vi "SineWave_testMyrioCounter.vi"() -> ()   [LabVIEW 2015]
uses:
  <vilib>/userdefined/High Color/nirio_resource_hc.ctl
  <vilib>/FPGAPlugInAG/myRIO-1900/niLvFpga_Open_myRIO-1900.vi
  <vilib>/FPGAPlugInAG/myRIO-1900/niLvFpga_Reset_myRIO-1900.vi
  <vilib>/rvi/interface/common/niFpgaWaitOnOcc.vi
  <vilib>/Utility/error.llb/Error Cluster From Error Code.vi
  <vilib>/rvi/errors/niLvFpgaAdjustHostInterfaceError.vi
  <vilib>/FPGAPlugInAG/myRIO-1900/niLvFpga_Run_myRIO-1900.vi
  <vilib>/FPGAPlugInAG/myRIO-1900/niLvFpga_Close_myRIO-1900.vi
  <vilib>/rvi/interface/nirviOpenFPGA/nirviOpenFPGA.xnode
  FPGA Bitfiles/MEMSPAMMyRIO_FPGATarget_testMyrioCounter_ZhKD5kzzM-g.lvbitx
  testMyrioCounter.vi
  <vilib>/rvi/interface/nirviMethod/nirviMethod.xnode
  <vilib>/rvi/interface/nirviReadWriteControl/nirviReadWriteControl.xnode
  <vilib>/rvi/interface/nirviCloseFPGA/nirviCloseFPGA.xnode
  <vilib>/Analysis/NI_AALPro.lvlib
  <vilib>/rvi/errors/niLvFpgaMergeErrorWithErrorCode.vi
  <vilib>/FPGAPlugInAG/myRIO-1900/niLvFpga_ConfigureFifo_myRIO-1900.vi
  <vilib>/FPGAPlugInAG/myRIO-1900/niLvFpga_WriteFifo_myRIO-1900.vi
  NiFpgaLv.dll
panel:
  out "Timed Out?":bool
  in  "stop":bool
  out "DA points":i32=440
  out "Bscan_Steps":u32[](graph)
  in  "Sample Num":u32=160
  in  "Range (V)":dbl=2.0 format="%0.2f"
  in  "Offset (V)":dbl format="%0.4f"
  in  "Phase0(deg)":dbl format="%0.2f"
  out "Vocie-coil Traj":i16[](graph)=[0, 16, 32, 48, 64, 80, 96, 111, 127, 142, 157, 171, 186, 200, 214, 228, 241, 254, 266, 278, 290, 301, 311, 322, 331, 341, 349, 357, 365, 372, 378, 384, 390, 394, 398, 402, 405, 407, 408, 409, 410, 409, 408, 407, 405, 402, 398, 394, 390, 384, 378, 372, 365, 357, 349, 341, 331, 322, 311, 301, 290, 278, 266, 254, 241, 228, 214, 200, 186, 171, 157, 142, 127, 111, 96, 80, 64, 48, 32, 16, 0, -16, -32, -48, -64, -80, -96, -111, -127, -142, -157, -171, -186, -200, -214, -228, -241, -254, -266, -278, -290, -301, -311, -322, -331, -341, -349, -357, -365, -372, -378, -384, -390, -394, -398, -402, -405, -407, -408, -409, -410, -409, -408, -407, -405, -402, -398, -394, -390, -384, -378, -372, -365, -357, -349, -341, -331, -322, -311, -301, -290, -278, -266, -254, -241, -228, -214, -200, -186, -171, -157, -142, -127, -111, -96, -80, -64, -48, -32, -16]
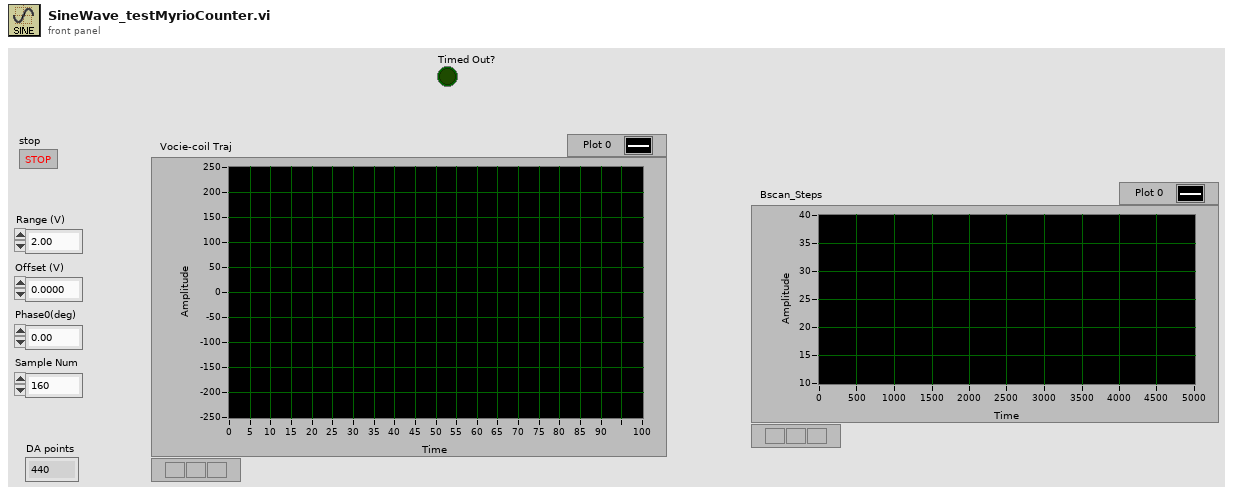
[diagram p1: front panel]
types:
  T1 = enum16{"sine", "cosine", "triangle", "square", "sawtooth", "increasing ramp", "decreasing ramp"}
  T2 = typedef "nirio_resource_hc.ctl" = tag
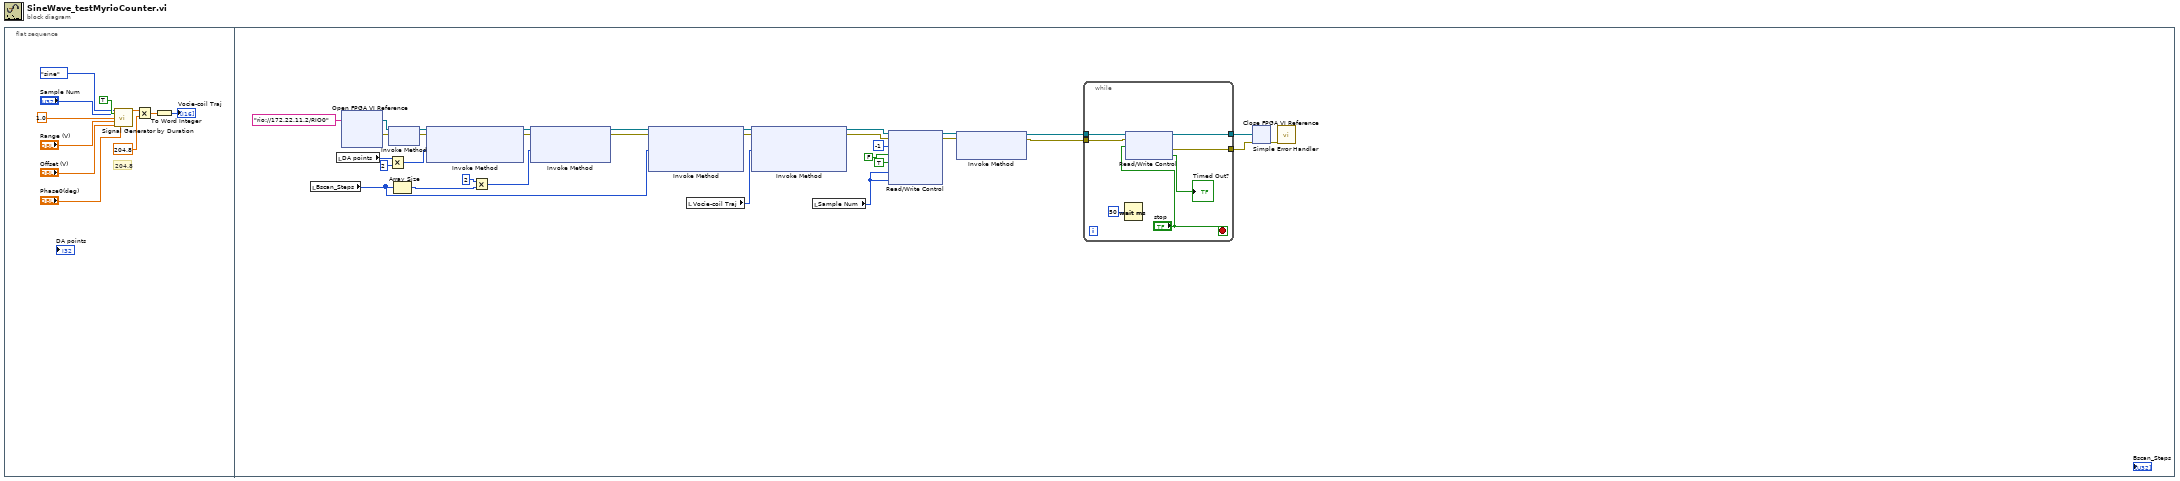
[diagram p0: block diagram]
diagram:
  n1 = flat-sequence {
    frame #0 {
      # "204.8"
      n2 = call <vilib>:"Signal Generator by Duration.vi"("signal type"=T1."sine", "reset phase"=TRUE, "# of samples"="Sample Num", "frequency"=1.0, "amplitude"="Range (V)", "dc offset"="Offset (V)", "phase in"="Phase0(deg)") -> ("signal"=w11:dbl[])  [unwired: 5 in, 3 out]
      n3 = Multiply(x=w11, y=204.8 ("frequency")) -> (x*y=w3:dbl[])
      n4 = To Word Integer(number=w3) -> (16bit integer=→"Vocie-coil Traj":i16[])
    }
    frame #1 {
      n5 = local read "Bscan_Steps"() -> (w40:u32[])
      n6 = local read "DA points"() -> (w15:i32)
      n7 = xnode "Open FPGA VI Reference"("resource name"=T2 "rio://172.22.11.2/RIO0") -> ("FPGA VI Reference Out"=w31:refnum<k20>, "error out"=w30:errorcluster)  [unwired: 1 in]
      n8 = xnode "Invoke Method"("FPGA VI Reference In"=w31, "error in"=w30) -> ("FPGA VI Reference Out"=w29:refnum<k20>, "error out"=w28:errorcluster)
      n9 = Multiply(x=w15, y=2) -> (x*y=w14:i32)
      n10 = Array Size(array=w40) -> (size(s)=w41:i32)
      n11 = xnode "Invoke Method"("FPGA VI Reference In"=w29, "error in"=w28, "Requested Depth"=w14) -> ("FPGA VI Reference Out"=w43:refnum<k20>, "error out"=w42:errorcluster)  [unwired: 1 out]
      n12 = Multiply(x=2, y=w41) -> (x*y=w37:i32)
      n13 = xnode "Invoke Method"("FPGA VI Reference In"=w43, "error in"=w42, "Requested Depth"=w37) -> ("FPGA VI Reference Out"=w34:refnum<k20>, "error out"=w33:errorcluster)  [unwired: 1 out]
      n14 = xnode "Invoke Method"("FPGA VI Reference In"=w34, "error in"=w33, "Data"=w40) -> ("FPGA VI Reference Out"=w35:refnum<k20>, "error out"=w36:errorcluster)  [unwired: 1 in, 1 out]
      n15 = local read "Vocie-coil Traj"() -> (w39:i16[])
      n16 = xnode "Invoke Method"("FPGA VI Reference In"=w35, "error in"=w36, "Data"=w39) -> ("FPGA VI Reference Out"=w27:refnum<k20>, "error out"=w24:errorcluster)  [unwired: 1 in, 1 out]
      n17 = local read "Sample Num"() -> (w12:u32)
      n18 = xnode "Read/Write Control"("FPGA VI Reference In"=w27, "error in"=w24, "FIFO_Timeout"=-1, "stop"=FALSE, "Sine"=TRUE, "VC_pt_in_fifo"=w12, "Trigperscan"=w12) -> ("FPGA VI Reference Out"=w25:refnum<k20>, "error out"=w23:errorcluster)
      n19 = xnode "Invoke Method"("FPGA VI Reference In"=w25, "error in"=w23) -> ("FPGA VI Reference Out"=w22:refnum<k20>, "error out"=w21:errorcluster)  [unwired: 1 in]
      n20 = while {
        tunnel: w22 -> [w49]
        tunnel: w21 -> [w48]
        tunnel: [w47] -> w19
        tunnel: [w46] -> w18
        stop <- "stop" stop-if-true
        n21 = Wait (ms)(milliseconds to wait=u32 50) -> ()  [unwired: 1 out]
        n22 = xnode "Read/Write Control"("FPGA VI Reference In"=w49, "error in"=w48, "stop"="stop") -> ("FPGA VI Reference Out"=w47:refnum<k20>, "error out"=w46:errorcluster, "Timed Out?"=→"Timed Out?":bool)
      }
      n23 = xnode "Close FPGA VI Reference"("FPGA VI Reference In"=w19, "error in"=w18) -> ("error out"=w20:errorcluster)
      n24 = call <vilib>:"Simple Error Handler.vi"("error in (no error)"=w20) -> ()  [unwired: 4 in, 5 out]
    }
  }
